vi "JoystickGlobals.vi"() -> ()   [LabVIEW 2015]
panel:
  out "JoystickValues":dbl[](array[numeric])
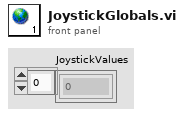
[diagram p1: front panel]
diagram:
